vi "Move sequencewithobstacle.vi"() -> ()   [LabVIEW 2021]
uses:
  <vilib>/myRIO/Instrument Drivers/Onboard IO/DIO/typedefs/DIO Reference.ctl
  <vilib>/myRIO/Common/Instrument Driver Framework/Utilities/typedefs/myRIO Generic Hardware Reference.ctl
  <vilib>/myRIO/Common/Instrument Driver Framework/Utilities/typedefs/Hardware Version Enum.ctl
  <vilib>/myRIO/Common/Instrument Driver Framework/Utilities/typedefs/myRIO v1.0 Reference.ctl
  <vilib>/myRIO/Common/Instrument Driver Framework/Utilities/typedefs/Generic FPGA Reference.ctl
  <vilib>/myRIO/Common/Instrument Driver Framework/myRIO v1.0/DIO/typedefs/DIO Channels List.ctl
  <vilib>/myRIO/Common/Instrument Driver Framework/myRIO v1.0/DIO/typedefs/DIO Channels Enum.ctl
  <vilib>/userdefined/High Color/nirio_resource_hc.ctl
  <vilib>/myRIO/Instrument Drivers/Onboard IO/PWM/typedefs/PWM Reference.ctl
  <vilib>/myRIO/Common/Instrument Driver Framework/myRIO v1.0/PWM/typedefs/PWM Channels Enum.ctl
  <vilib>/myRIO/Instrument Drivers/Onboard IO/PWM/typedefs/PWM Configuration.ctl
  <vilib>/myRIO/Common/Instrument Driver Framework/Utilities/vis/Is FPGA Ref Available.vi
  <vilib>/myRIO/Common/Instrument Driver Framework/myRIO v1.0/DIO/vis/myRIO v1.1 Open DIO.vi
  <vilib>/myRIO/Instrument Drivers/Onboard IO/DIO/vis/Read.vi
  <vilib>/myRIO/Common/Instrument Driver Framework/myRIO v1.0/PWM/vis/myRIO v1.1 Open PWM.vi
  <vilib>/myRIO/Instrument Drivers/Onboard IO/PWM/vis/Set Duty Cycle and Frequency.vi
  <vilib>/myRIO/Instrument Drivers/Onboard IO/DIO/vis/Write.vi
  <vilib>/myRIO/Common/Instrument Driver Framework/Utilities/vis/Validate Channels.vi
  <vilib>/myRIO/Common/Instrument Driver Framework/myRIO v1.0/DIO/vis/myRIO v1.0 Reserve DIO.vi
  <vilib>/myRIO/Common/Instrument Driver Framework/myRIO v1.0/PWM/vis/myRIO v1.0 Reserve PWM.vi
  <vilib>/myRIO/Common/Instrument Driver Framework/myRIO v1.0/UART/vis/myRIO v1.0 Close UART.vi
  <vilib>/myRIO/Common/Instrument Driver Framework/myRIO v1.0/Resource Manager/vis/myRIO v1.0 Reserve Channel List.vi
  <vilib>/myRIO/Common/Instrument Driver Framework/myRIO v1.0/DIO/vis/myRIO v1.0 Build MUX Configuration DIO.vi
  <vilib>/myRIO/Common/Instrument Driver Framework/myRIO v1.0/PWM/vis/myRIO v1.0 Build MUX Configuration PWM.vi
  <vilib>/myRIO/Common/Instrument Driver Framework/myRIO v1.0/Resource Manager/vis/myRIO v1.0 Reserve Channel.vi
  <vilib>/myRIO/Common/Instrument Driver Framework/myRIO v1.0/Resource Manager/vis/myRIO v1.0 Unreserve Channel.vi
  <vilib>/myRIO/Common/Instrument Driver Framework/myRIO v1.0/Resource Manager/vis/myRIO v1.0 Create Configuration List.vi
  <vilib>/myRIO/Common/Instrument Driver Framework/myRIO v1.0/Resource Manager/vis/myRIO v1.0 Build Mutex Name.vi
  <vilib>/robotics/Navigation/shared/MapNode/OccupancyGridNode/NI_Robotics_OccupancyGridMapNode.lvclass
  C:/Program Files (x86)/National Instruments/LabVIEW 2021/vi.lib/robotics/Navigation/shared/MapNode/AbstractAstarNode/NI_Robotics_AbstractAstarNode.lvclass
  <vilib>/robotics/Navigation/shared/WorldMap/OccupancyGridWorldMap/NI_Robotics_OccupancyGridWorldMap.lvclass
  C:/Program Files (x86)/National Instruments/LabVIEW 2021/vi.lib/robotics/Navigation/shared/WorldMap/AbstractWorldMap/NI_Robotics_AbstractWorldMap.lvclass
  <vilib>/Utility/VariantDataType/GetNumericInfo.vi
  <vilib>/Utility/error.llb/Error Cluster From Error Code.vi
  <vilib>/myRIO/Common/Instrument Driver Framework/myRIO v1.0/myRIO v1.1 Open.vi
  <vilib>/myRIO/Common/Instrument Driver Framework/Utilities/vis/IO Manager.vi
  <vilib>/myRIO/Common/Instrument Driver Framework/Utilities/vis/Configuration Manager.vi
  <vilib>/myRIO/Common/Instrument Driver Framework/myRIO v1.0/Resource Manager/vis/myRIO v1.0 Configure IO.vi
  <vilib>/myRIO/Common/Instrument Driver Framework/myRIO v1.0/myRIO v1.0 Close.vi
  <vilib>/myRIO/Common/Instrument Driver Framework/myRIO v1.0/DIO/vis/myRIO v1.0 Read DIO.vi
  <vilib>/myRIO/Common/Instrument Driver Framework/myRIO v1.0/PWM/vis/myRIO v1.0 Write PWM.vi
  <vilib>/myRIO/Common/Instrument Driver Framework/myRIO v1.0/DIO/vis/myRIO v1.0 Write DIO.vi
  <vilib>/myRIO/Common/Instrument Driver Framework/Utilities/vis/FPGA Ref Manager.vi
  <vilib>/myRIO/Common/Instrument Driver Framework/myRIO v1.0/myRIO v1.0 Reset FPGA.vi
  <vilib>/myRIO/Common/Instrument Driver Framework/myRIO v1.0/IRQ/vis/myRIO v1.0 IRQ Info FGV.vi
  <vilib>/myRIO/Common/Instrument Driver Framework/myRIO v1.0/IRQ/vis/myRIO v1.0 Timer IRQ Info FGV.vi
  <vilib>/myRIO/Common/Instrument Driver Framework/myRIO v1.0/IRQ/vis/myRIO v1.0 ISR Agent.vi
  <vilib>/myRIO/Instrument Drivers/Utilities/vis/Reset Index.vi
  <vilib>/myRIO/Common/Instrument Driver Framework/myRIO v1.0/Resource Manager/vis/myRIO v1.0 Block Write Resource Manager.vi
  <vilib>/myRIO/Express VI/Onboard Devices/Button/Button Express VI.xnode
  <vilib>/myRIO/Instrument Drivers/Onboard IO/DIO/vis/myRIO DIO Open.xnode
  <vilib>/myRIO/Express VI/Onboard IO/PWM/PWM Express VI.xnode
  <vilib>/myRIO/Instrument Drivers/Onboard IO/PWM/vis/myRIO PWM Open.xnode
  <vilib>/myRIO/Express VI/Onboard Devices/LED/LED Express VI.xnode
  <vilib>/myRIO/Instrument Drivers/Utilities/Utilities.lvlib
  <vilib>/myRIO/Instrument Drivers/Onboard IO/PWM/PWM.lvlib
  <vilib>/myRIO/Instrument Drivers/Onboard IO/DIO/DIO.lvlib
  <vilib>/robotics/Navigation/NI_Robotics_Navigation .lvlib
panel:
  out "loop \ncount":i32
  in  "y start":i32
  in  "x start":i32
  out "Next coordinate (x)":i32
  out "Next coordinate(y)":i32
  out "Intensity Graph":dbl[][](graph)
  in  "Condition":dbl
  out "yyyy":i32
  out "xxxxx 2":i32
  in  "x end stop":i32
  in  "y end stop":i32
  in  "Next path step":i32=1
  in  "2D array":dbl[][](array[numeric])
  in  "stop":bool
  # "2  no obstacle"
  # "0 obstacle in Y"
  # "1 obstacle  x"
  # "-1 obstacle -x"
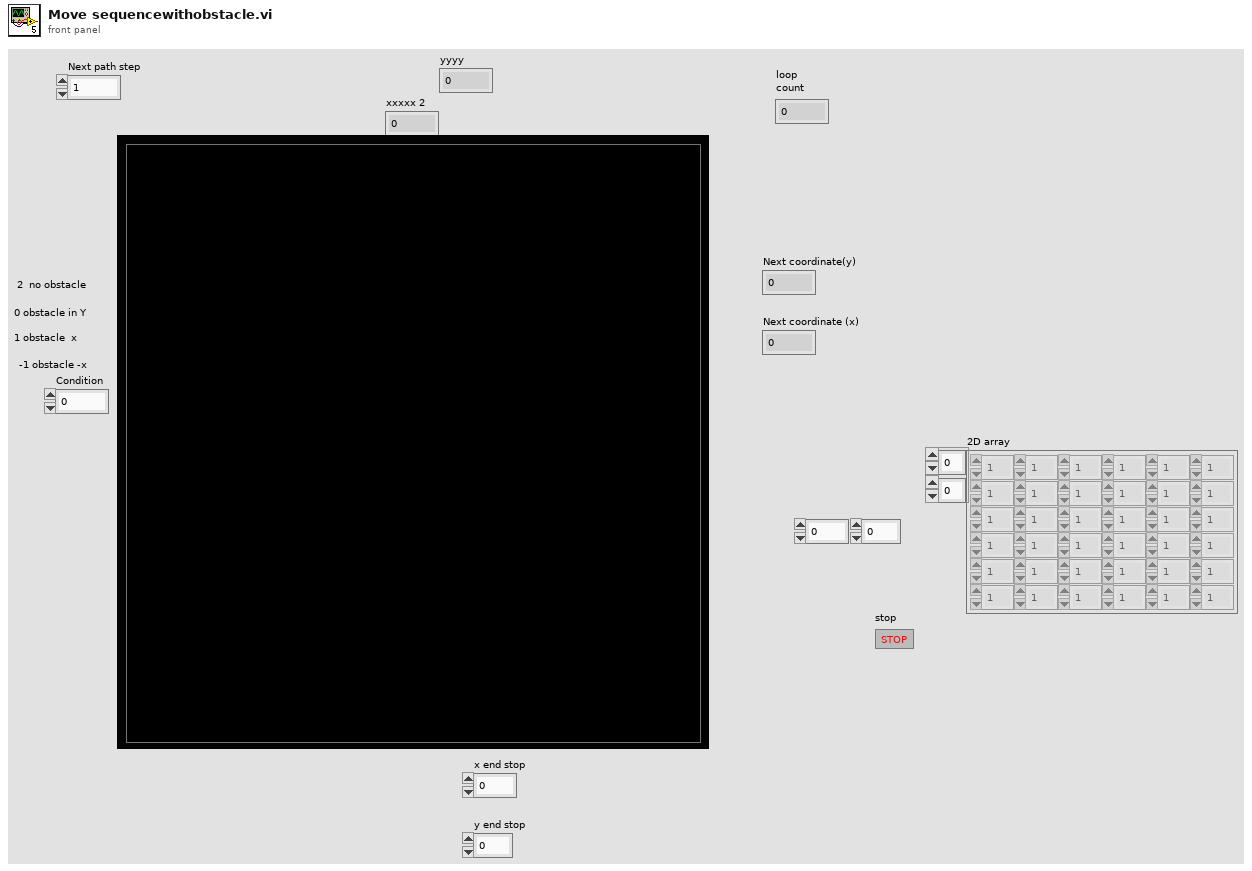
[diagram p1: front panel]
types:
  T1 = typedef "DIO.lvlib/DIO Reference.ctl" = cluster{"myRIO Reference":T2, "DIO Channels List":T6}
  T2 = typedef "myRIO Generic Hardware Reference.ctl" = cluster{"myRIO Model":T3, "myRIO Hardware Reference":T4}
  T3 = typedef "Hardware Version Enum.ctl" = enum16{"Unknown", "myRIO-1900", "myRIO-1950", "roboRIO", "NI ELVIS RIO CM", "ELVIS III"}
  T4 = typedef "myRIO v1.0 Reference.ctl" = cluster{"Generic FPGA Reference":T5, "Allow multiple opens":bool}
  T5 = typedef "Generic FPGA Reference.ctl" = refnum<k20>
  T6 = typedef "DIO Channels List.ctl" = T7[]
  T7 = typedef "DIO Channels Enum.ctl" = enum16{"Not Connected", "C/DIO0", "C/DIO1", "C/DIO2", "C/DIO3", "C/DIO4", "C/DIO5", "C/DIO6", "C/DIO7", "A/DIO0", "A/DIO1", "A/DIO2", "A/DIO3", "A/DIO4", "A/DIO5", "A/DIO6", "A/DIO7", "A/DIO8", "A/DIO9", "A/DIO10", "A/DIO11", "A/DIO12", "A/DIO13", "A/DIO14", "A/DIO15", "A/DIO16", "A/DIO17", "A/DIO18", "A/DIO19", "B/DIO0", "B/DIO1", "B/DIO2", "B/DIO3", "B/DIO4", "B/DIO5", "B/DIO6", "B/DIO7", "B/DIO8", "B/DIO9", "B/DIO10", "B/DIO11", "B/DIO12", "B/DIO13", "B/DIO14", "B/DIO15", "B/DIO16", "B/DIO17", "B/DIO18", "B/DIO19", "LED0", "LED1", "LED2", "LED3", "Button0", "DIO/DIO0", "DIO/DIO1", "DIO/DIO2", "DIO/DIO3", "DIO/DIO4", "DIO/DIO5", "DIO/DIO6", "DIO/DIO7", "DIO/DIO8", "DIO/DIO9", "SPI/CS0", "SPI/CS1", "SPI/CS2", "SPI/CS3", "LED RADIO (Green)", "LED RADIO (Red)", "LED COMM (Green)", "LED COMM (Red)", "LED MODE (Green)", "LED MODE (Red)"}
  T8 = typedef "nirio_resource_hc.ctl" = tag
  T9 = typedef "PWM.lvlib/PWM Reference.ctl" = cluster{"myRIO Reference":T2, "PWM Channels Enum":T10, "PWM Configuration":T11}
  T10 = typedef "PWM Channels Enum.ctl" = enum16{"Not Connected", "C/PWM0", "C/PWM1", "A/PWM0", "A/PWM1", "A/PWM2", "A/PWM3", "A/PWM4", "A/PWM5", "A/PWM6", "A/PWM7", "A/PWM8", "A/PWM9", "A/PWM10", "A/PWM11", "A/PWM12", "A/PWM13", "A/PWM14", "A/PWM15", "A/PWM16", "A/PWM17", "A/PWM18", "A/PWM19", "B/PWM0", "B/PWM1", "B/PWM2", "B/PWM3", "B/PWM4", "B/PWM5", "B/PWM6", "B/PWM7", "B/PWM8", "B/PWM9", "B/PWM10", "B/PWM11", "B/PWM12", "B/PWM13", "B/PWM14", "B/PWM15", "B/PWM16", "B/PWM17", "B/PWM18", "B/PWM19", "PWM/PWM0", "PWM/PWM1", "PWM/PWM2", "PWM/PWM3", "PWM/PWM4", "PWM/PWM5", "PWM/PWM6", "PWM/PWM7", "PWM/PWM8", "PWM/PWM9"}
  T11 = typedef "PWM.lvlib/PWM Configuration.ctl" = cluster{"Frequency":dbl, "Duty Cycle":dbl}
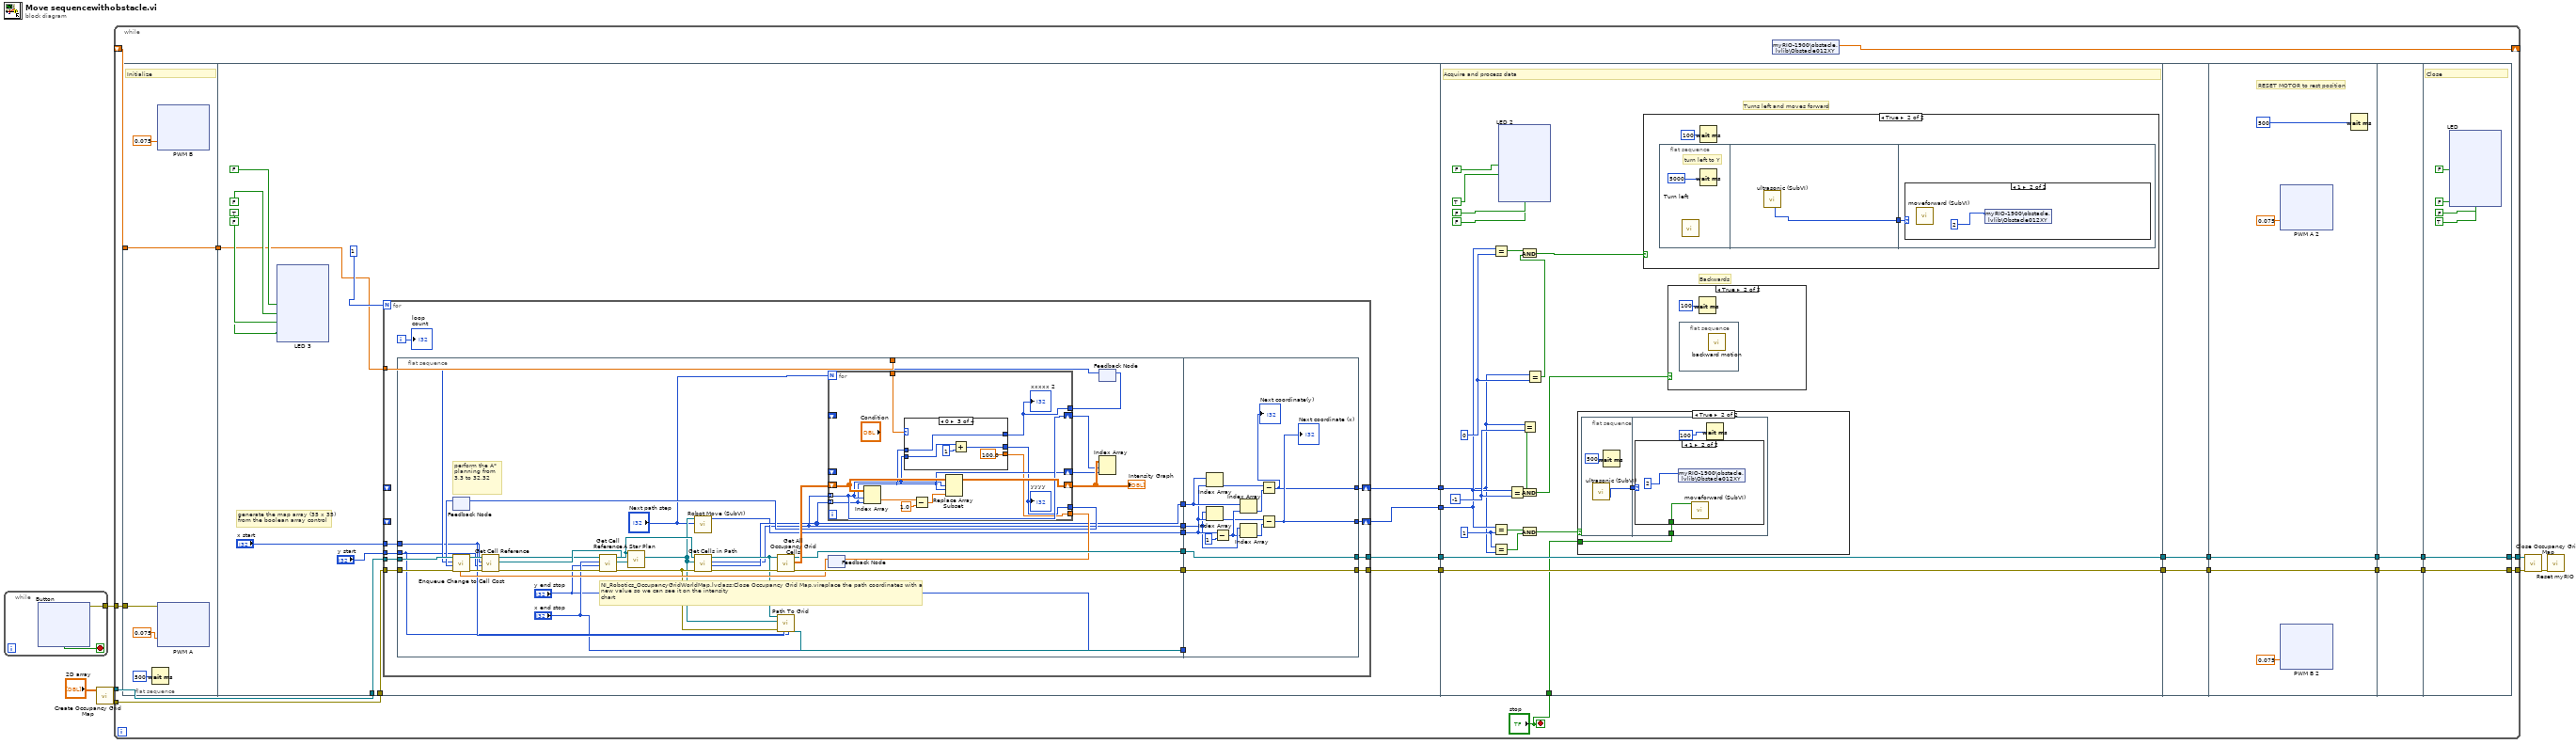
[diagram p0: block diagram]
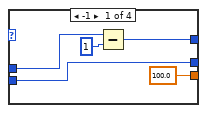
[diagram p2: hidden frame]
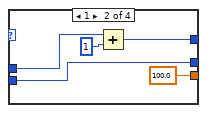
[diagram p3: hidden frame]
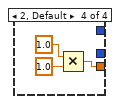
[diagram p4: hidden frame]
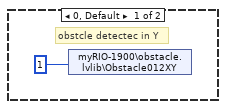
[diagram p7: hidden frame]
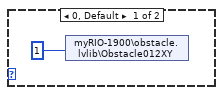
[diagram p9: hidden frame]
diagram:
  n1 = while {
    tunnel: [w8] -> w1
    stop <- w9 stop-if-true
    n2 = xnode "Button"() -> ("Value"=w9:bool, "error out"=w8:errorcluster)  [unwired: 1 in]
  }
  n3 = call <vilib>:"Create Occupancy Grid Map.vi"("occupancy grid"="2D array") -> ("error out"=w3:errorcluster, "map reference out"=w2:refnum<data-value>)  [unwired: 9 in]
  n4 = while {
    tunnel: [w53] -> w6
    tunnel: [w52] -> w5
    tunnel: w3 -> [w51]
    tunnel: w2 -> [w50]
    tunnel: w1 -> [w49]
    shift-right: [w45] -> _
    shift-left: _ -> [w46]
    stop <- "stop" stop-if-true
    n5 = flat-sequence {
      tunnel: w49 -> [w67]
      tunnel: [w66] -> w47
      tunnel: w46 -> [w66]
      tunnel: [w152] -> w65
      tunnel: [w151] -> w64
      tunnel: [w150] -> w57
      tunnel: [w149] -> w56
      tunnel: w51 -> [w147]
      tunnel: w50 -> [w146]
      tunnel: w47 -> [w141]
      tunnel: w65 -> [w296]
      tunnel: w64 -> [w295]
      tunnel: [w296] -> w61
      tunnel: [w295] -> w58
      tunnel: w57 -> [w294]
      tunnel: w56 -> [w293]
      tunnel: "stop" -> [w288]
      tunnel: [w366] -> w62
      tunnel: w61 -> [w366]
      tunnel: [w365] -> w59
      tunnel: w58 -> [w365]
      tunnel: [w368] -> w63
      tunnel: w62 -> [w368]
      tunnel: [w367] -> w60
      tunnel: w59 -> [w367]
      tunnel: w63 -> [w443]
      tunnel: w60 -> [w442]
      tunnel: [w443] -> w55
      tunnel: [w442] -> w54
      tunnel: w55 -> [w449]
      tunnel: w54 -> [w448]
      tunnel: [w449] -> w53
      tunnel: [w448] -> w52
      frame #0 {
        # "Initialize"
        n6 = Wait (ms)(milliseconds to wait=u32 500) -> ()  [unwired: 1 out]
        n7 = xnode "PWM B"("Duty Cycle"=0.075) -> ()  [unwired: 1 in, 1 out]
        n8 = xnode "PWM A"("Duty Cycle"=0.075, "error in (no error)"=w67) -> ()  [unwired: 1 out]
      }
      frame #1 {
        # "generate the map array (35 x 35)\nfrom the boolean array control"
        n9 = xnode "LED 3"("LED3"=FALSE, "LED1"=FALSE, "LED2"=TRUE, "LED0"=FALSE) -> ()  [unwired: 1 in, 1 out]
        n10 = for {
          N: 1 -> [_]
          tunnel: [w210] -> w151
          tunnel: [w209] -> w152
          tunnel: "x start" -> [w206]
          tunnel: "y start" -> [w205]
          shift-right: [w204] -> w150
          shift-left: _ -> [_]
          shift-right: [w199] -> w149
          shift-left: _ -> [_]
          tunnel: w147 -> [w196]
          tunnel: w146 -> [w195]
          tunnel: w141 -> [w193]
          i -> [w194]
          n11 = flat-sequence {
            tunnel: w196 -> [w236]
            tunnel: w195 -> [w235]
            tunnel: [w234] -> w208
            tunnel: [w233] -> w207
            tunnel: w206 -> [w222]
            tunnel: w205 -> [w221]
            tunnel: [w217] -> w203
            tunnel: [w216] -> w202
            tunnel: [w215] -> w201
            tunnel: [w214] -> w200
            tunnel: ["x end stop"] -> w198
            tunnel: ["y end stop"] -> w197
            tunnel: w193 -> [w211]
            tunnel: [w286] -> w209
            tunnel: [w287] -> w210
            tunnel: w208 -> [w287]
            tunnel: w207 -> [w286]
            tunnel: [w282] -> w204
            tunnel: [w281] -> w199
            tunnel: w203 -> [w285]
            tunnel: w202 -> [w284]
            tunnel: w201 -> [w283]
            tunnel: w200 -> [_]
            tunnel: w198 -> [_]
            tunnel: w197 -> [_]
            frame #0 {
              # "NI_Robotics_OccupancyGridWorldMap.lvclass:Close Occupancy Grid Map.vireplace the path coordinates with a\nnew value so we can see it on the intensity \nchart"
              # "perform the A* planning from 3,3 to 32,32"
              n12 = feedback #1() -> (w229:i32)  [unwired: 1 in]
              n13 = feedback #2() -> (w226:dbl)  [unwired: 1 in]
              n14 = feedback #3() -> (w228:i32)  [unwired: 1 in]
              n15 = call <vilib>:"Enqueue Change to Cell Cost.vi"("cost"=w226, "error in (no error)"=w236, "y"=w229, "x"=w228, "map reference in"=w235) -> ("error out"=w237:errorcluster, "map reference out"=w238:refnum<data-value>)  [unwired: 5 in]
              n16 = call <vilib>:"Get Cell Reference.vi"("error in (no error)"=w237, "y"=w221, "x"=w222, "map reference in"=w238) -> ("error out"=w239:errorcluster, "cell reference"=w242:refnum<data-value>, "map reference out"=w240:refnum<data-value>)  [unwired: 4 in, 1 out]
              n17 = call <vilib>:"Get Cell Reference.vi"("error in (no error)"=w239, "y"="y end stop", "x"="x end stop", "map reference in"=w240) -> ("error out"=w223:errorcluster, "cell reference"=w241:refnum<data-value>, "map reference out"=w245:refnum<data-value>)  [unwired: 4 in, 1 out]
              n18 = call <vilib>:"A Star Plan.vi"("goal reference"=w241, "start reference"=w242, "map reference in"=w245) -> ("path references"=w220:refnum<data-value>[])  [unwired: 5 in, 3 out]
              n19 = call "Robot Move (SubVI).vi"("Move Robot in"="Next path step", "path references"=w220) -> ("Move Robot 3"=w216:i32)  [unwired: 9 in]
              n20 = call <vilib>:"Get Cells in Path.vi"("error in (no error)"=w223, "path references"=w220, "map reference in"=w245) -> ("error out"=w243:errorcluster, "y coordinates"=w217:i32[], "x coordinates"=w215:i32[], "map reference out"=w224:refnum<data-value>)  [unwired: 5 in]
              n21 = call <vilib>:"Get All Occupancy Grid Cells.vi"("error in (no error)"=w243, "map reference in"=w224) -> ("error out"=w233:errorcluster, "occupancy grid"=w244:dbl[][], "map reference out"=w234:refnum<data-value>)  [unwired: 7 in]
              n22 = call "Path To Grid.vi"("current y"=w221, "current x"=w222, "error in (no error)"=w223, "path references"=w220, "map reference in"=w224) -> ("map reference out"=w214:refnum<data-value>)  [unwired: 2 in, 4 out]
              n23 = for {
                N: "Next path step" -> [_]
                tunnel: w217 -> [w250] mode=indexing
                tunnel: w215 -> [w251] mode=indexing
                shift-right: [w256] -> w232
                shift-left: w244 -> [w253]
                shift-right: [w250] -> w230
                shift-left: _ -> [_]
                shift-right: [w251] -> w231
                shift-left: _ -> [_]
                tunnel: [w249] -> w227
                tunnel: [w248] -> w219
                tunnel: [w247] -> w225
                tunnel: w211 -> [w246]
                n24 = Index Array(array=w253, index (row)=w251, index (col)=w250) -> (element=w252:dbl)
                n25 = case shown="0" w246 {
                  tunnel: w251 -> [w257 w262 w271 _]
                  tunnel: [w257 w262 w269 _] -> w248
                  tunnel: w250 -> [w261 w265 w267 _]
                  tunnel: [w260 w264 w267 _] -> w247
                  tunnel: [100.0 100.0 100.0 w274] -> w249
                  frame -1 {
                    n26 = Subtract(x=w261, y=1) -> (x-y=w260:i32)
                  }
                  frame 1 {
                    n27 = Add(x=w265, y=1) -> (x+y=w264:i32)
                  }
                  frame 0 {
                    n28 = Add(x=w271, y=1) -> (x+y=w269:i32)
                  }
                  frame 2, Default {
                    n29 = Multiply(x=1.0, y=1.0) -> (x*y=w274:dbl)
                  }
                }
                "yyyy" <- w248
                "xxxxx 2" <- w247
                n30 = Subtract(x=w252, y=1.0) -> (x-y=w255:dbl)
                n31 = Replace Array Subset(array=w253, new element=w255, index (row)=w251, index (col)=w250) -> (w256:dbl[][])
              }
              "Intensity Graph" <- w232
              n32 = feedback-in #1(w219) -> ()
              n33 = feedback-in #2(w227) -> ()
              n34 = feedback-in #3(w225) -> ()
              n35 = Index Array(array=w232, index (row)=w231, index (col)=w230) -> ()  [unwired: 1 out]
            }
            frame #1 {
              n36 = Index Array(array=w285, index=w284) -> (element=w277:i32)
              n37 = Index Array(array=w283, index=w284) -> (element=w278:i32)
              n38 = Subtract(x=w284, y=1) -> (x-y=w279:i32)
              n39 = Index Array(array=w285, index=w279) -> (element=w275:i32)
              n40 = Index Array(array=w283, index=w279) -> (element=w276:i32)
              n41 = Subtract(x=w277, y=w275) -> (x-y=w281:i32)
              "Next coordinate(y)" <- w281
              n42 = Subtract(x=w278, y=w276) -> (x-y=w282:i32)
              "Next coordinate (x)" <- w282
            }
          }
          "loop \ncount" <- w194
        }
      }
      frame #2 {
        w302 = -1
        w305 = 0
        w308 = 1
        # "Backwards"
        # "Turns left and moves forward"
        # "Acquire and process data"
        n43 = Equal?(x=w294, y=w305) -> (x = y?=w304:bool)
        n44 = Equal?(x=w294, y=w308) -> (x = y?=w307:bool)
        n45 = Equal?(x=w308, y=w293) -> (x = y?=w306:bool)
        n46 = xnode "LED 2"("LED3"=FALSE, "LED1"=TRUE, "LED2"=FALSE, "LED0"=FALSE) -> ()  [unwired: 1 in, 1 out]
        n47 = Equal?(x=w294, y=w302) -> (x = y?=w300:bool)
        n48 = Equal?(x=w293, y=w302) -> (x = y?=w301:bool)
        n49 = And(x=w301, y=w300) -> (x .and. y?=w297:bool)
        n50 = And(x=w307, y=w306) -> (x .and. y?=w299:bool)
        n51 = Equal?(x=w293, y=w305) -> (x = y?=w303:bool)
        n52 = And(x=w304, y=w303) -> (x .and. y?=w298:bool)
        n53 = case shown="True" w299 {
          tunnel: w288 -> [_ w356]
          frame False {
          }
          frame True {
            n54 = flat-sequence {
              tunnel: [w357] -> w355
              tunnel: w356 -> [w361]
              tunnel: w355 -> [w359]
              frame #0 {
                n55 = call "ultrasonic (SubVI).vi"() -> ("0, 1"=w357:i16)  [unwired: 9 in, 2 out]
                n56 = Wait (ms)(milliseconds to wait=u32 500) -> ()  [unwired: 1 out]
              }
              frame #1 {
                n57 = case shown="1" w359 {
                  tunnel: w361 -> [_ w364]
                  frame 0, Default {
                    n58 = shared-variable "myRIO-1900\\obstacle.lvlib\\Obstacle012XY"(1) -> ()  [unwired: 1 in, 1 out]
                  }
                  frame 1 {
                    n59 = shared-variable "myRIO-1900\\obstacle.lvlib\\Obstacle012XY"(2) -> ()  [unwired: 1 in, 1 out]
                    n60 = call "moveforward (SubVI).vi"("Stop Button"=w364) -> ()  [unwired: 7 in, 4 out]
                  }
                }
                n61 = Wait (ms)(milliseconds to wait=u32 100) -> ()  [unwired: 1 out]
              }
            }
          }
        }
        n62 = case shown="True" w298 {
          frame False {
          }
          frame True {
            n63 = flat-sequence {
              tunnel: [w351] -> w348
              tunnel: w348 -> [w352]
              frame #0 {
                # "turn left to Y"
                n64 = call "Turn left.vi"() -> ()  [unwired: 8 in, 4 out]
                n65 = Wait (ms)(milliseconds to wait=u32 5000) -> ()  [unwired: 1 out]
              }
              frame #1 {
                n66 = call "ultrasonic (SubVI).vi"() -> ("0, 1"=w351:i16)  [unwired: 9 in, 2 out]
              }
              frame #2 {
                n67 = case shown="1" w352 {
                  frame 0, Default {
                    # "obstcle detectec in Y"
                    n68 = shared-variable "myRIO-1900\\obstacle.lvlib\\Obstacle012XY"(1) -> ()  [unwired: 1 in, 1 out]
                  }
                  frame 1 {
                    n69 = call "moveforward (SubVI).vi"() -> ()  [unwired: 8 in, 4 out]
                    n70 = shared-variable "myRIO-1900\\obstacle.lvlib\\Obstacle012XY"(2) -> ()  [unwired: 1 in, 1 out]
                  }
                }
              }
            }
            n71 = Wait (ms)(milliseconds to wait=u32 100) -> ()  [unwired: 1 out]
          }
        }
        n72 = case shown="True" w297 {
          frame False {
          }
          frame True {
            n73 = flat-sequence {
              frame #0 {
                n74 = call "backward motion.vi"() -> ()  [unwired: 12 in]
              }
            }
            n75 = Wait (ms)(milliseconds to wait=u32 100) -> ()  [unwired: 1 out]
          }
        }
      }
      frame #3 {
      }
      frame #4 {
        # "RESET MOTOR to rest position"
        n76 = xnode "PWM A 2"("Duty Cycle"=0.075) -> ()  [unwired: 1 in, 1 out]
        n77 = xnode "PWM B 2"("Duty Cycle"=0.075) -> ()  [unwired: 1 in, 1 out]
        n78 = Wait (ms)(milliseconds to wait=u32 500) -> ()  [unwired: 1 out]
      }
      frame #5 {
      }
      frame #6 {
        # "Close"
        n79 = xnode "LED"("LED3"=FALSE, "LED1"=FALSE, "LED2"=FALSE, "LED0"=TRUE) -> ()  [unwired: 1 in, 1 out]
      }
    }
    n80 = shared-variable "myRIO-1900\\obstacle.lvlib\\Obstacle012XY"() -> (w45:dbl)  [unwired: 1 in, 1 out]
  }
  n81 = call <vilib>:"Close Occupancy Grid Map.vi"("error in (no error)"=w6, "map reference in"=w5) -> ("error out"=w7:errorcluster)  [unwired: 9 in]
  n82 = call <vilib>:"Reset myRIO.vi"("error in (no error)"=w7) -> ()  [unwired: 10 in, 1 out]
